vi "TSM Set DAQmx Tasks.vi"(0 "TSM context":T1) -> (15 "error out":errorcluster)   [LabVIEW 2019]
doc: "Use this VI to initialize AI and AO tasks for all NI-DAQmx instruments in the pin map associated with the test program."
uses:
  <vilib>/NI_TestStand_SemiconductorModule/NI_TestStand_Semiconductor_Module.lvlibp/PinMap/General/SemiconductorModuleContext.ctl
  <vilib>/DAQmx/create/channels.llb/DAQmx Create Channel (AI-Voltage-Basic).vi
  <vilib>/DAQmx/create/channels.llb/DAQmx Create Channel (AO-Voltage-Basic).vi
  <vilib>/DAQmx/create/channels.llb/DAQmx Create Channel (DO-Digital Output).vi
  <vilib>/NI_TestStand_SemiconductorModule/NI_TestStand_Semiconductor_Module.lvlibp
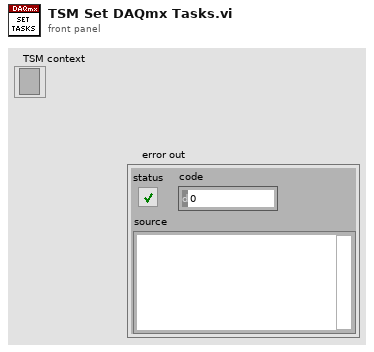
[diagram p1: front panel]
types:
  T1 = typedef "NI_TestStand_Semiconductor_Module.lvlibp/SemiconductorModuleContext.ctl" = refnum<k7>
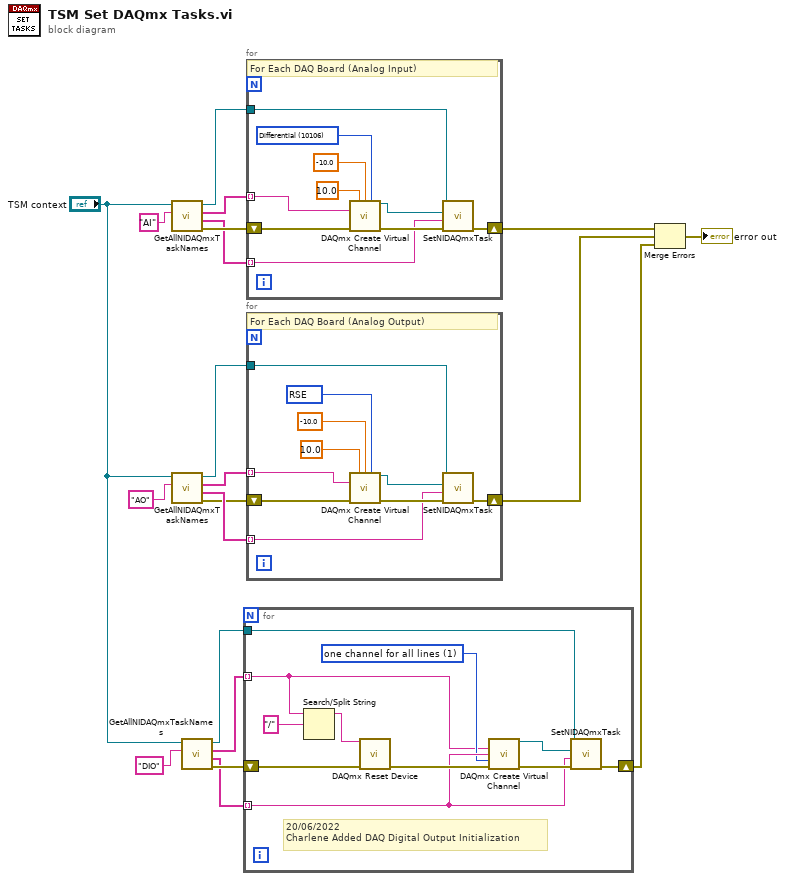
[diagram p0: block diagram]
diagram:
  n1 = call <vilib>:"GetAllNIDAQmxTaskNames.vi"("Task Type"="AI", "Semiconductor Module Context"="TSM context") -> ("error out"=w18:errorcluster, "Task Names"=w17:string[], "Channel Lists"=w16:string[], "Semiconductor Module Context Out"=w20:T1)  [unwired: 6 in]
  n2 = call <vilib>:"GetAllNIDAQmxTaskNames.vi"("Task Type"="AO", "Semiconductor Module Context"="TSM context") -> ("error out"=w11:errorcluster, "Task Names"=w12:string[], "Channel Lists"=w13:string[], "Semiconductor Module Context Out"=w10:T1)  [unwired: 6 in]
  n3 = call <vilib>:"GetAllNIDAQmxTaskNames.vi"("Task Type"="DIO", "Semiconductor Module Context"="TSM context") -> ("error out"=w6:errorcluster, "Task Names"=w4:string[], "Channel Lists"=w5:string[], "Semiconductor Module Context Out"=w2:T1)  [unwired: 6 in]
  n4 = for {
    shift-right: [w29] -> w1
    shift-left: w6 -> [w31]
    tunnel: w5 -> [w21] mode=indexing
    tunnel: w4 -> [w25] mode=indexing
    tunnel: w2 -> [w23]
    w22 = 1 items=["one channel for each line", "one channel for all lines"] ("line grouping")
    # "20/06/2022\nCharlene Added DAQ Digital Output Initialization"
    n5 = Search/Split String(string=w21, search string/char (-)="/") -> (substring before match=w26:string)  [unwired: 1 in, 2 out]
    n6 = call <vilib>:"DAQmx Reset Device.vi"("device in"=w26, "error in"=w31) -> ("error out"=w30:errorcluster)  [unwired: 13 in]
    n7 = call-poly <vilib>:"DAQmx Create Virtual Channel.vi"("lines"=w21, "name to assign"=w25, "line grouping"=w22, "error in"=w30) -> ("task out"=w24:refnum<k21>, "error out"=w28:errorcluster)  [unwired: 10 in]
    n8 = call <vilib>:"SetNIDAQmxTask.vi"("error in (no error)"=w28, "Task Name"=w25, "DAQmx Task"=w24, "Semiconductor Module Context"=w23) -> ("error out"=w29:errorcluster)  [unwired: 6 in, 1 out]
  }
  n9 = for {
    tunnel: w20 -> [w40]
    tunnel: w17 -> [w32] mode=indexing
    tunnel: w16 -> [w36] mode=indexing
    shift-right: [w37] -> w19
    shift-left: w18 -> [w41]
    w35 = 10106 items=["default"=-1, "RSE"=10083, "NRSE"=10078, "Differential"=10106, "Pseudodifferential"=12529] ("input terminal configuration")
    # "For Each DAQ Board (Analog Input)"
    n10 = call-poly <vilib>:"DAQmx Create Virtual Channel.vi"("maximum value"=10.0, "minimum value"=-10.0, "input terminal configuration"=w35, "physical channels"=w36, "error in"=w41) -> ("task out"=w39:refnum<k21>, "error out"=w38:errorcluster)  [unwired: 9 in]
    n11 = call <vilib>:"SetNIDAQmxTask.vi"("error in (no error)"=w38, "Task Name"=w32, "DAQmx Task"=w39, "Semiconductor Module Context"=w40) -> ("error out"=w37:errorcluster)  [unwired: 6 in, 1 out]
  }
  n12 = for {
    tunnel: w10 -> [w50]
    tunnel: w12 -> [w42] mode=indexing
    tunnel: w13 -> [w46] mode=indexing
    shift-right: [w47] -> w8
    shift-left: w11 -> [w51]
    w45 = 10083 items=["default"=-1, "RSE"=10083, "NRSE"=10078, "Differential"=10106, "Pseudodifferential"=12529] ("input terminal configuration")
    # "For Each DAQ Board (Analog Output)"
    n13 = call-poly <vilib>:"DAQmx Create Virtual Channel.vi"("maximum value"=10.0, "minimum value"=-10.0, "output terminal configuration"=w45, "physical channels"=w46, "error in"=w51) -> ("task out"=w49:refnum<k21>, "error out"=w48:errorcluster)  [unwired: 9 in]
    n14 = call <vilib>:"SetNIDAQmxTask.vi"("error in (no error)"=w48, "Task Name"=w42, "DAQmx Task"=w49, "Semiconductor Module Context"=w50) -> ("error out"=w47:errorcluster)  [unwired: 6 in, 1 out]
  }
  n15 = Merge Errors(w19, w8, w1) -> (→"error out":errorcluster)
